vi "Test - Draw Teapot.vi"() -> ()   [LabVIEW 2020, in "Raster.lvlib"]
uses:
  Raster.lvlib
  Utility/Utility.lvlib
  Rectangle Dimensions.ctl
  5ea285c7-be76-47ab-bb95-511c6a9aac96.vi
  d84cddbd-8e40-43c7-a758-6e8d8fd6f2c6.vi
  Graphics Global (For Debug).vi
  3D/Vector 3D.ctl
  3D/3D.lvlib
  UV.ctl
  3D/Vertex.ctl
  3D/Triangle.ctl
  Texture.ctl
  3D/Material.ctl
panel:
  out "Pixel count":u32
  in  "Teapot":T1[](array[typedef]) {"Vertex 3"."UV"."v" min=0 max=1 step=0.1; "Vertex 3"."UV"."u" min=0 max=1 step=0.1; "Vertex 2"."UV"."v" min=0 max=1 step=0.1; "Vertex 2"."UV"."u" min=0 max=1 step=0.1; "Vertex 1"."UV"."v" min=0 max=1 step=0.1; "Vertex 1"."UV"."u" min=0 max=1 step=0.1}
  out "Time [s]":dbl format="%.3p"
  out "new picture":picture
  # "(0,0)"
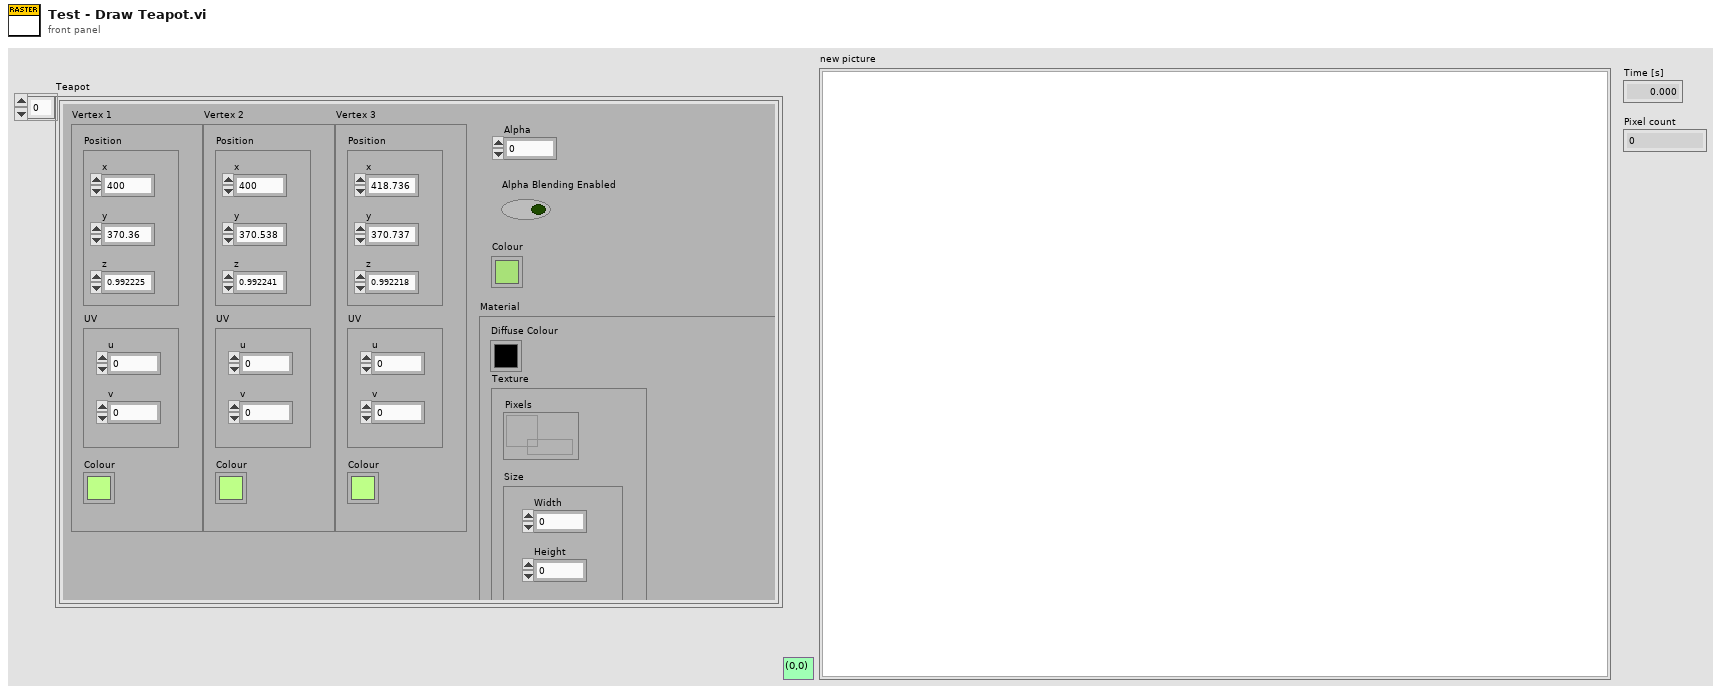
[diagram p1: front panel]
types:
  T1 = typedef "3D.lvlib/Triangle.ctl" = cluster{"Vertex 1":T2, "Vertex 2":T2, "Vertex 3":T2, "Alpha":dbl, "Alpha Blending Enabled":bool, "Colour":u32, "Material":T5}
  T2 = typedef "3D.lvlib/Vertex.ctl" = cluster{"Position":T3, "UV":T4, "Colour":u32}
  T3 = typedef "3D.lvlib/Vector 3D.ctl" = cluster{"x":sgl, "y":sgl, "z":sgl}
  T4 = typedef "Raster.lvlib/UV.ctl" = cluster{"u":sgl, "v":sgl}
  T5 = typedef "3D.lvlib/Material.ctl" = cluster{"Diffuse Colour":u32, "Texture":T6}
  T6 = typedef "Raster.lvlib/Texture.ctl" = cluster{"Pixels":refnum<data-value>, "Size":T7}
  T7 = typedef "Raster.lvlib/Rectangle Dimensions.ctl" = cluster{"Width":u32, "Height":u32}
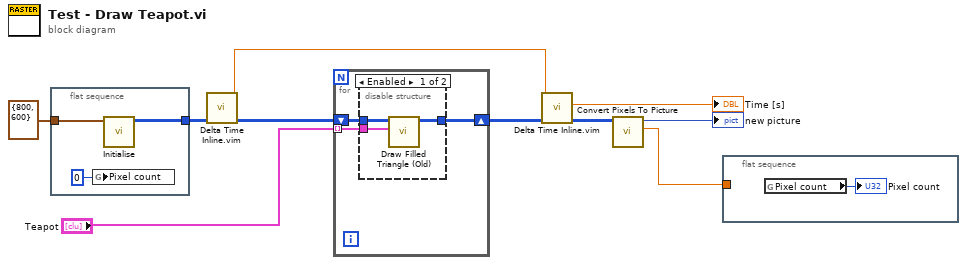
[diagram p0: block diagram]
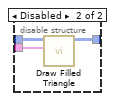
[diagram p2: hidden frame]
diagram:
  n1 = flat-sequence {
    tunnel: T7 {"Width"=800, "Height"=600} ("Screen Dimensions") -> [w13]
    tunnel: [w12] -> w8
    frame #0 {
      n2 = global write "Graphics Global (For Debug).vi" "Pixel count"(u32 0 ("Pixel count")) -> ()
      n3 = call "Initialise.vi"("Screen Dimensions"=w13) -> ("Pixel Data out"=w12:u32[][])  [unwired: 10 in]
    }
  }
  n4 = call "Delta Time Inline.vim"("value in"=w8) -> ("value out"=w7:u32[][], "Relative Seconds out [s]"=w3:dbl)  [unwired: 8 in, 1 out]
  n5 = for {
    tunnel: "Teapot" -> [w14] mode=indexing
    shift-right: [w15] -> w6
    shift-left: w7 -> [w16]
    n6 = disable-structure shown="Enabled" {
      disable-tunnel: w16 -> [w19 w22]
      disable-tunnel: [w18 w21] -> w15
      disable-tunnel: w14 -> [w17 w20]
      frame Enabled {
        n7 = call "Draw Filled Triangle (Old).vi"("Triangle"=w17, "Pixel Data in"=w19) -> ("Pixel Data out"=w18:u32[][])  [unwired: 9 in]
      }
      frame Disabled {
        n8 = call "Draw Filled Triangle.vi"("Triangle"=w20, "Pixel Data in"=w22) -> ("Pixel Data out"=w21:u32[][])  [unwired: 9 in]
      }
    }
  }
  n9 = call "Delta Time Inline.vim"("value in"=w6, "Relative Seconds in [s]"=w3) -> ("value out"=w5:u32[][], "Delta Time [s]"=→"Time [s]":dbl)  [unwired: 7 in, 1 out]
  n10 = call "Convert Pixels To Picture.vi"("Pixel Data in"=w5) -> ("Present Time [s]"=w1:dbl, "2D Picture"=→"new picture":picture)  [unwired: 9 in]
  n11 = flat-sequence {
    tunnel: w1 -> [_]
    frame #0 {
      n12 = global read "Graphics Global (For Debug).vi" "Pixel count"() -> (→"Pixel count":u32)
    }
  }
